vi "Calculate Metrics.vi"(7 "Error Percentage":dbl, 8 "Error In":errorcluster, 9 "INL Method":T1=enum."End Point", 10 "Input Values":T3, 11 "Application In":refnum<class "Application.lvclass">) -> (0 "Error Out":errorcluster, 1 "Transfer Function":T2, 2 "DNL Values":dbl[](array[numeric]), 3 "Application Out":refnum<class "Application.lvclass">, 5 "INL Values":dbl[](array[numeric]))   [LabVIEW 2023, in "Application.lvclass"]
uses:
  Application.lvclass
  Typedef/Input Values.ctl
  Typedef/Transfer Function.ctl
  Typedef/INL Method.ctl
  Mode/Mode.lvclass
  C:/Users/Ancy.Augustin/Downloads/INL DNL/INL DNL/Classes/Application/Application.lvclass
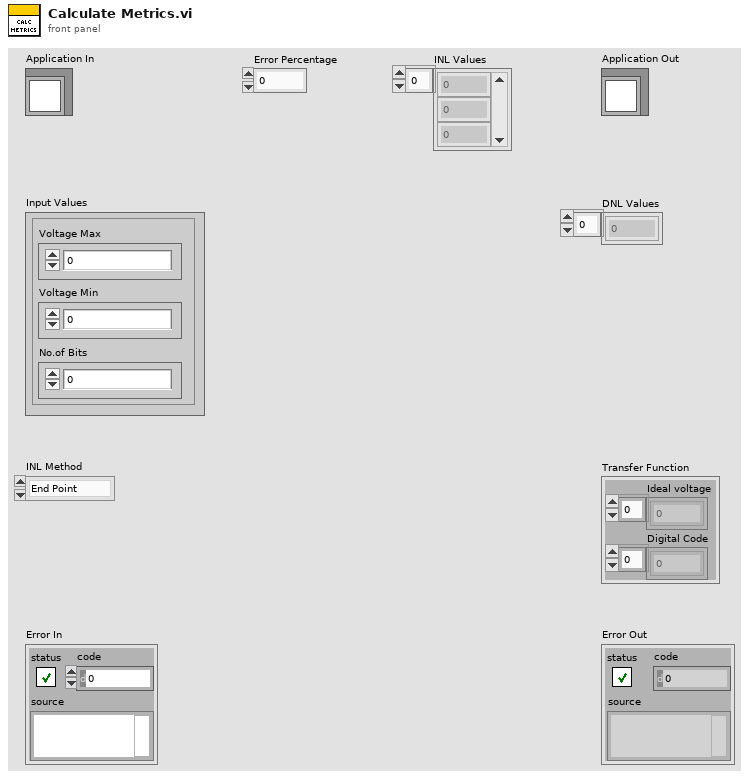
[diagram p1: front panel]
types:
  T1 = typedef "INL Method.ctl" = enum16{"Best Fit", "End Point"}
  T2 = typedef "Transfer Function.ctl" = cluster{"Ideal voltage":dbl[], "Digital Code":dbl[]}
  T3 = typedef "Input Values.ctl" = cluster{"Voltage Max":dbl, "Voltage Min":dbl, "No.of Bits":i32}
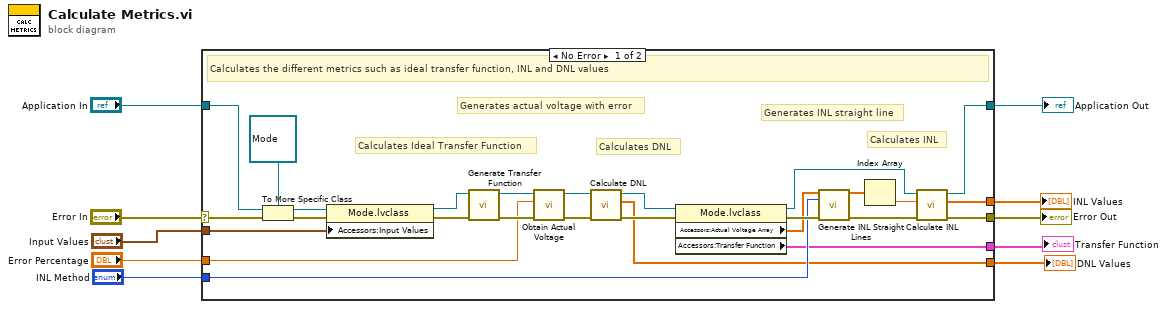
[diagram p0: block diagram]
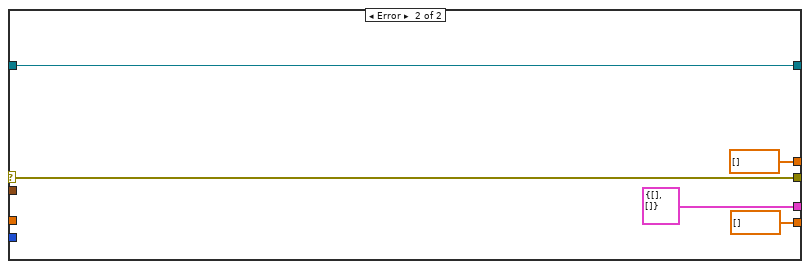
[diagram p2: hidden frame]
diagram:
  n1 = case shown="No Error" "Error In" {
    selector: "Error In" -> [w37 w42]
    tunnel: [w18 w42] -> w9
    tunnel: "Input Values" -> [w30 _]
    tunnel: [w13 dbl[] [] ("DNL")] -> w7
    tunnel: [w12 dbl[] [] ("INL")] -> w6
    tunnel: "INL Method" -> [w19 _]
    tunnel: "Application In" -> [w34 w38]
    tunnel: "Error Percentage" -> [w26 _]
    tunnel: [w14 T2 {"Ideal voltage"=[], "Digital Code"=[]} ("Accessors:Transfer Function")] -> w2
    tunnel: [w11 w38] -> w1
    frame No Error {
      # "Calculates INL"
      # "Generates INL straight line"
      # "Calculates DNL"
      # "Generates actual voltage with error"
      # "Calculates Ideal Transfer Function"
      # "Calculates the different metrics such as ideal transfer function, INL and DNL values"
      n2 = To More Specific Class(target class=refnum<class "Mode.lvclass"> refnum ("Mode.lvclass"), reference=w34, error in=w37) -> (specific class reference=w31:refnum<class "Mode.lvclass">, error out=w35:errorcluster)
      n3 = property class="Mode.lvclass"(reference=w31, error in=w35, "Accessors:Input Values"=w30) -> (reference out=w29:refnum<class "Mode.lvclass">, error out=w32:errorcluster)
      n4 = call-dynamic "Generate Transfer Function.vi"("Error In"=w32, "Mode In"=w29) -> ("Error Out"=w36:errorcluster, "Mode Out"=w27:refnum<class "Mode.lvclass">)  [unwired: 8 in]
      n5 = call-dynamic "Obtain Actual Voltage.vi"("Error In"=w36, "Error Percentage"=w26, "Mode in"=w27) -> ("Error Out"=w28:errorcluster, "Mode out"=w23:refnum<class "Mode.lvclass">)  [unwired: 7 in]
      n6 = call-dynamic "Calculate DNL.vi"("Error In"=w28, "Mode in"=w23) -> ("Error Out"=w25:errorcluster, "DNL"=w13:dbl[], "Mode out"=w21:refnum<class "Mode.lvclass">)  [unwired: 7 in]
      n7 = property class="Mode.lvclass"(reference=w21, error in=w25) -> (reference out=w16:refnum<class "Mode.lvclass">, error out=w22:errorcluster, "Accessors:Actual Voltage Array"=w20:dbl[], "Accessors:Transfer Function"=w14:T2)
      n8 = call "Generate INL Straight Lines.vi"("Actual Transfer Function"=w20, "INL Method"=w19, "Error In"=w22) -> ("Straight Line"=w17:dbl[], "Error Out"=w24:errorcluster)  [unwired: 11 in]
      n9 = Index Array(array=w17) -> (element=w15:dbl)  [unwired: 1 in]
      n10 = call-dynamic "Calculate INL.vi"("Error In"=w24, "V Zero"=w15, "Mode in"=w16) -> ("Error Out"=w18:errorcluster, "INL"=w12:dbl[], "Mode out"=w11:refnum<class "Mode.lvclass">)  [unwired: 6 in]
    }
    frame Error {
    }
  }
  "Error Out" <- w9
  "Transfer Function" <- w2
  "DNL Values" <- w7
  "INL Values" <- w6
  "Application Out" <- w1
